vi "MetodoInit.vi"(8 "error in (no error)":errorcluster, 11 "Osciloscope in":refnum<class "Osciloscope.lvclass">) -> (0 "error out":errorcluster, 3 "Osciloscope out":refnum<class "Osciloscope.lvclass">)   [LabVIEW 2020, in "Osciloscope.lvclass"]
uses:
  Osciloscope.lvclass
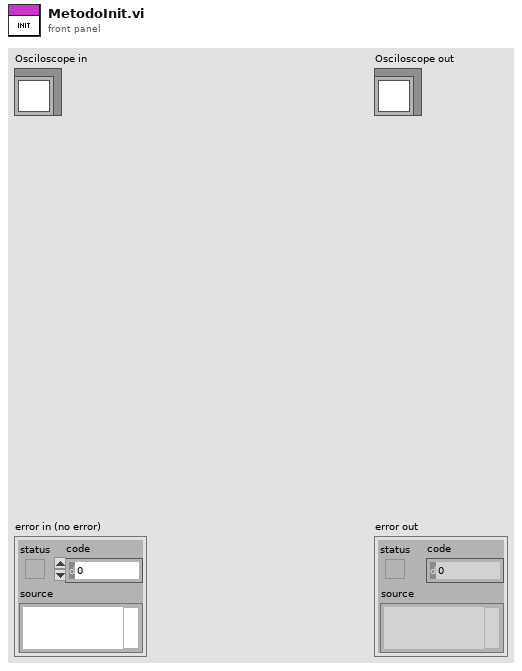
[diagram p1: front panel]
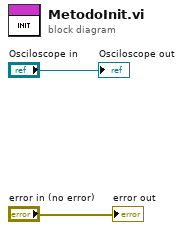
[diagram p0: block diagram]
diagram:
  "error out" <- "error in (no error)"
  "Osciloscope out" <- "Osciloscope in"
